vi "LinearSystemSim_setState.vi"(9 "System State":T1, 11 "in LinearSystemSim":T2) -> (0 "Size Coerced":bool, 3 "out LinearSystemSim":T2)   [LabVIEW 2019, in "Trajectory_Library.lvlib"]
doc: "Sets the system state.\n \nInputs:\n - LinearSystemSim -- Data cluster\n - SystemState -- The new state.\n\nOutputs:\n - OutLinearSystemSim -- Updated data cluster\n - SizeCoerced -- If TRUE, an error occured. Execution may continue."
uses:
  Trajectory_Library.lvlib
  TypeDef/LINEAR_SYSTEM.ctl
  <vilib>/Analysis/Matrix/Datatypes/RealMatrix.ctl
  <vilib>/Analysis/Matrix/NI_Matrix.lvlib
  TypeDef/LINEAR_SYSTEM_SIM.ctl
panel:
  # "<States, 1>"
  # "<Outputs, 1>"
  # "<Inputs, 1>"
  # "<Outputs, 1>"
  # "<States,States>"
  # "<States,Inputs>"
  # "<Outputs,States>"
  # "<Outputs,Inputs>"
  # "<States, 1>"
  # "<Outputs, 1>"
  # "<Inputs, 1>"
  # "<Outputs, 1>"
  # "<States,States>"
  # "<States,Inputs>"
  # "<Outputs,States>"
  # "<Outputs,Inputs>"
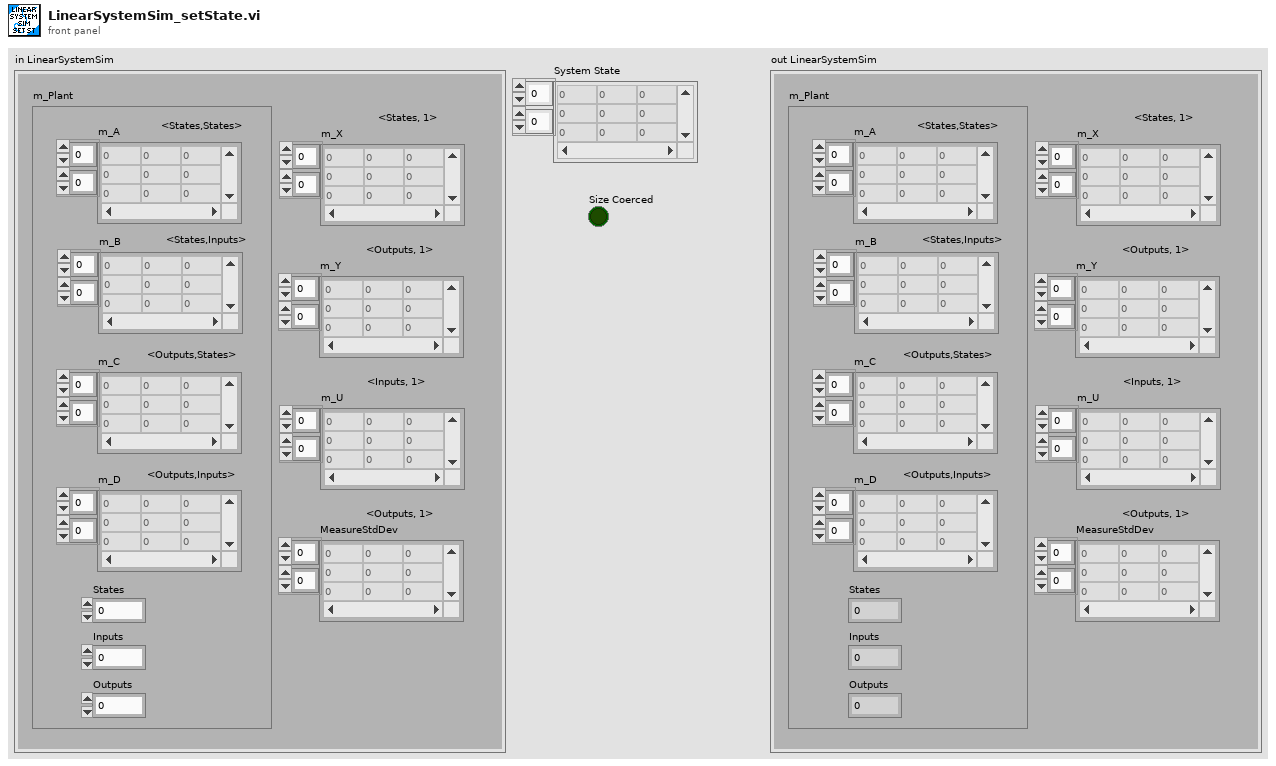
[diagram p1: front panel]
types:
  T1 = typedef "NI_Matrix.lvlib/RealMatrix.ctl" = dbl[][]
  T2 = typedef "Trajectory_Library.lvlib/LINEAR_SYSTEM_SIM.ctl" = cluster{"m_Plant":T3, "m_X":T1, "m_Y":T1, "m_U":T1, "MeasureStdDev":T1}
  T3 = typedef "Trajectory_Library.lvlib/LINEAR_SYSTEM.ctl" = cluster{"m_A":T1, "m_B":T1, "m_C":T1, "m_D":T1, "States":i32, "Inputs":i32, "Outputs":i32}
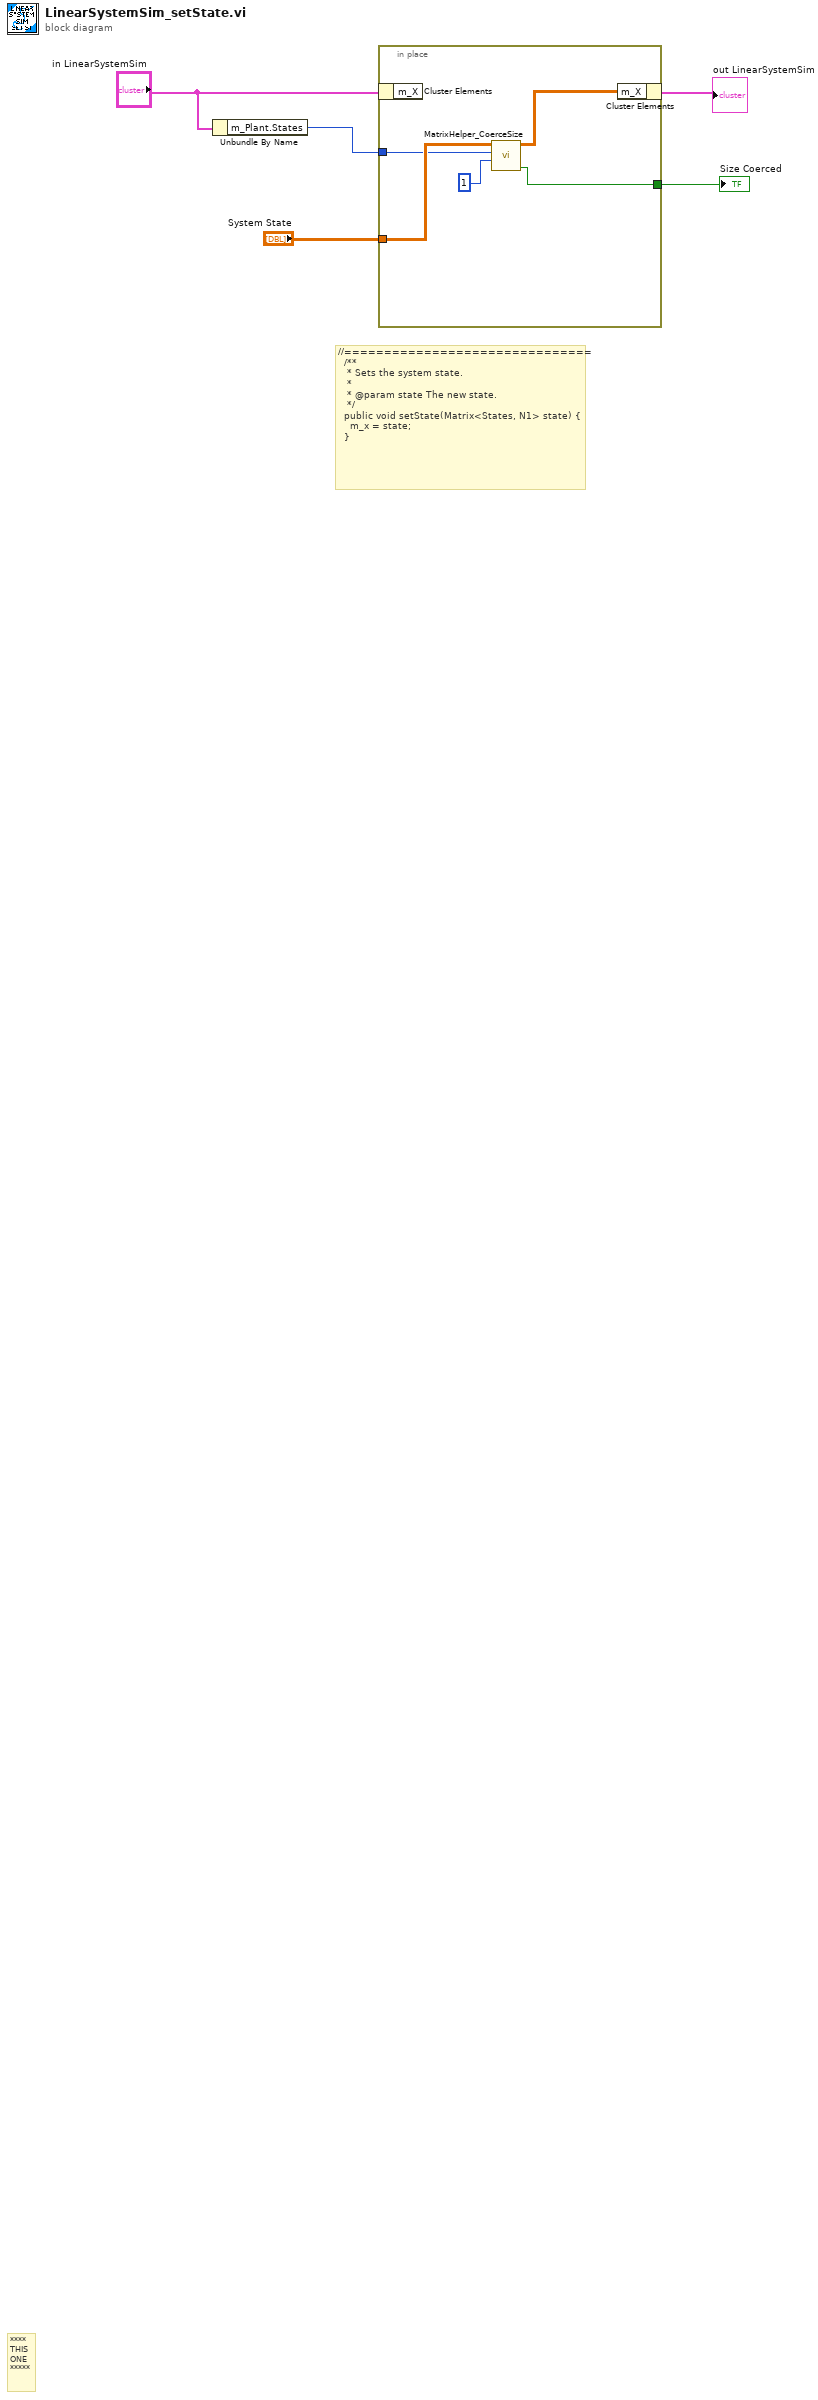
[diagram p0: block diagram]
diagram:
  # "//===============================\n  /**\n   * Sets the system state.\n   *\n   * @param state The new state.\n   */\n  public void setState(Matrix<States, N1> state) {\n    m_x = state;\n  }"
  # "****\nTHIS\nONE\n*****"
  n1 = Unbundle By Name("in LinearSystemSim") -> ("m_Plant.States"=w2:i32)
  n2 = in-place {
    in-place-border: "System State" -> [w10]
    in-place-border: w2 -> [w8]
    in-place-border: [w6] -> w1
    n3 = in-place-cluster #1("in LinearSystemSim") -> ()  [unwired: 1 out]
    n4 = call "MatrixHelper_CoerceSize.vi"("Columns"=1, "Rows"=w8, "input matrix"=w10) -> ("Coerced"=w6:bool, "output matrix"=w7:T1)  [unwired: 7 in]
    n5 = in-place-cluster #1("m_X"=w7) -> (→"out LinearSystemSim":T2)
  }
  "Size Coerced" <- w1
